vi "ROS_Master_addToQueue.vi"(2 "Message":string, 3 "ROS_Master in":T1) -> ()   [LabVIEW 2016]
doc: "Adds a message to the queue"
uses:
  ROS_Master.ctl
  ROS_Topic.ctl
  ROS_Node.ctl
  ROS_Service.ctl
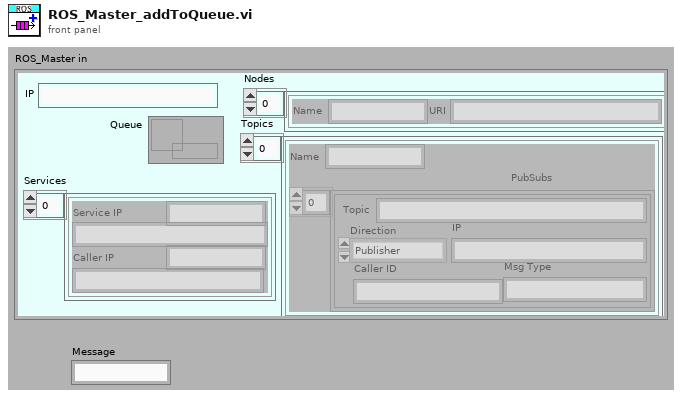
[diagram p1: front panel]
types:
  T1 = typedef "ROS_Master.ctl" = cluster{"IP":string, "Topics":cluster{"Name":string, "PubSubs":T2[]}[], "Nodes":T3[], "Services":T4[], "Queue":refnum<queue>}
  T2 = typedef "ROS_Topic.ctl" = cluster{"Caller ID":string, "IP":string, "Msg Type":string, "Direction":enum16{"Publisher", "Subscriber"}, "Topic":string}
  T3 = typedef "ROS_Node.ctl" = cluster{"Name":string, "URI":string}
  T4 = typedef "ROS_Service.ctl" = cluster{"Service":string, "Service IP":string, "Caller IP":string, "Caller ID":string}
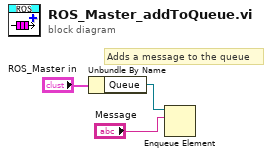
[diagram p0: block diagram]
diagram:
  # "Adds a message to the queue"
  n1 = Unbundle By Name("ROS_Master in") -> ("Queue"=w3:refnum<queue>)
  n2 = Enqueue Element(queue=w3, element="Message") -> ()  [unwired: 2 in, 3 out]
